vi "PC_Shot_PowerOG.vi"(5 "Bounce T/F?":bool, 7 "Puck Selection":enum32{"PTFE", "Nylon"}(radio), 8 "Error In":errorcluster, 11 "PC Data":T1) -> (0 "Error Out":errorcluster, 3 "Power %":dbl)   [LabVIEW 2017]
uses:
  pc_data.ctl
  <vilib>/vision/Image Controls.llb/IMAQ Image.ctl
  <vilib>/Utility/file.llb/Read Delimited Spreadsheet (DBL).vi
panel:
  out "Goal Y Straight":dbl
  in  "Friction PTFE":dbl=0.4
  in  "Puck Mass PTFE":dbl=0.0069
  in  "Friction Nylon":dbl=0.31
  in  "Puck Mass Nylon":dbl=0.0037
  out "mm/pixels":dbl
  out "Goal Y Bounce":dbl
  out "Wall X Bounce":dbl
  out "Pot Position":dbl
  out "Kicker angle":dbl
  in  "Pendulum length":dbl=0.069
  in  "Pendulum mass":dbl=0.096
  out "Required E":dbl
  in  "Kicker Res":dbl=0.5
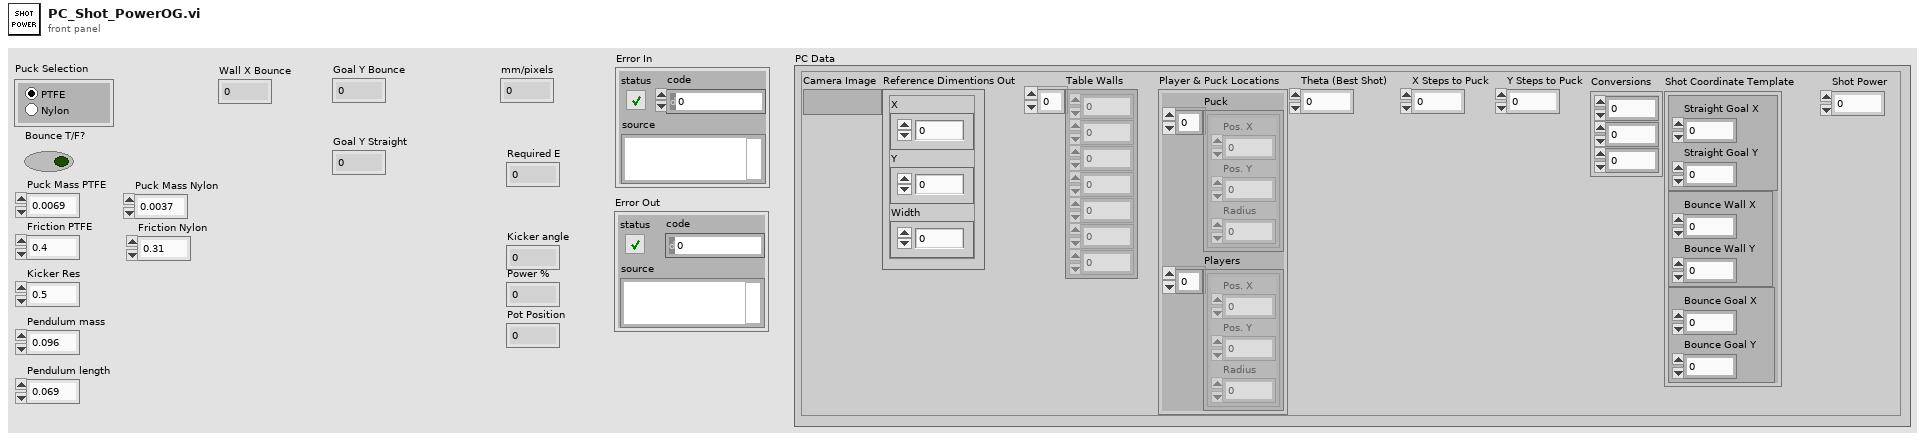
[diagram p1: front panel]
types:
  T1 = typedef "pc_data.ctl" = cluster{"Camera Image":T2, "Reference Dimentions Out":cluster{"X":dbl, "Y":dbl, "Width":dbl}, "Table Walls":sgl[], "Player & Puck Locations":cluster{"Puck":cluster{"Pos. X":i32, "Pos. Y":i32, "Radius":i32}[], "Players":cluster{"Pos. X":i32, "Pos. Y":i32, "Radius":i32}[]}, "Theta (Best Shot)":dbl, "X Steps to Puck":dbl, "Y Steps to Puck":dbl, "Conversions":cluster{dbl, dbl, dbl}, "Shot Coordinate Template":cluster{cluster{"Straight Goal X":sgl, "Straight Goal Y":dbl}, cluster{"Bounce Wall X":dbl, "Bounce Wall Y":sgl}, cluster{"Bounce Goal X":sgl, "Bounce Goal Y":dbl}}, "Shot Power":dbl}
  T2 = typedef "IMAQ Image.ctl" = refnum<image>
  T3 = cluster{"Pos. X":i32, "Pos. Y":i32, "Radius":i32}[]
  T4 = cluster{cluster{"Straight Goal X":sgl, "Straight Goal Y":dbl}, cluster{"Bounce Wall X":dbl, "Bounce Wall Y":sgl}, cluster{"Bounce Goal X":sgl, "Bounce Goal Y":dbl}}
  T5 = cluster{"Straight Goal X":sgl, "Straight Goal Y":dbl}
  T6 = cluster{"Bounce Wall X":dbl, "Bounce Wall Y":sgl}
  T7 = cluster{"Bounce Goal X":sgl, "Bounce Goal Y":dbl}
  T8 = cluster{"Pos. X":i32, "Pos. Y":i32, "Radius":i32}
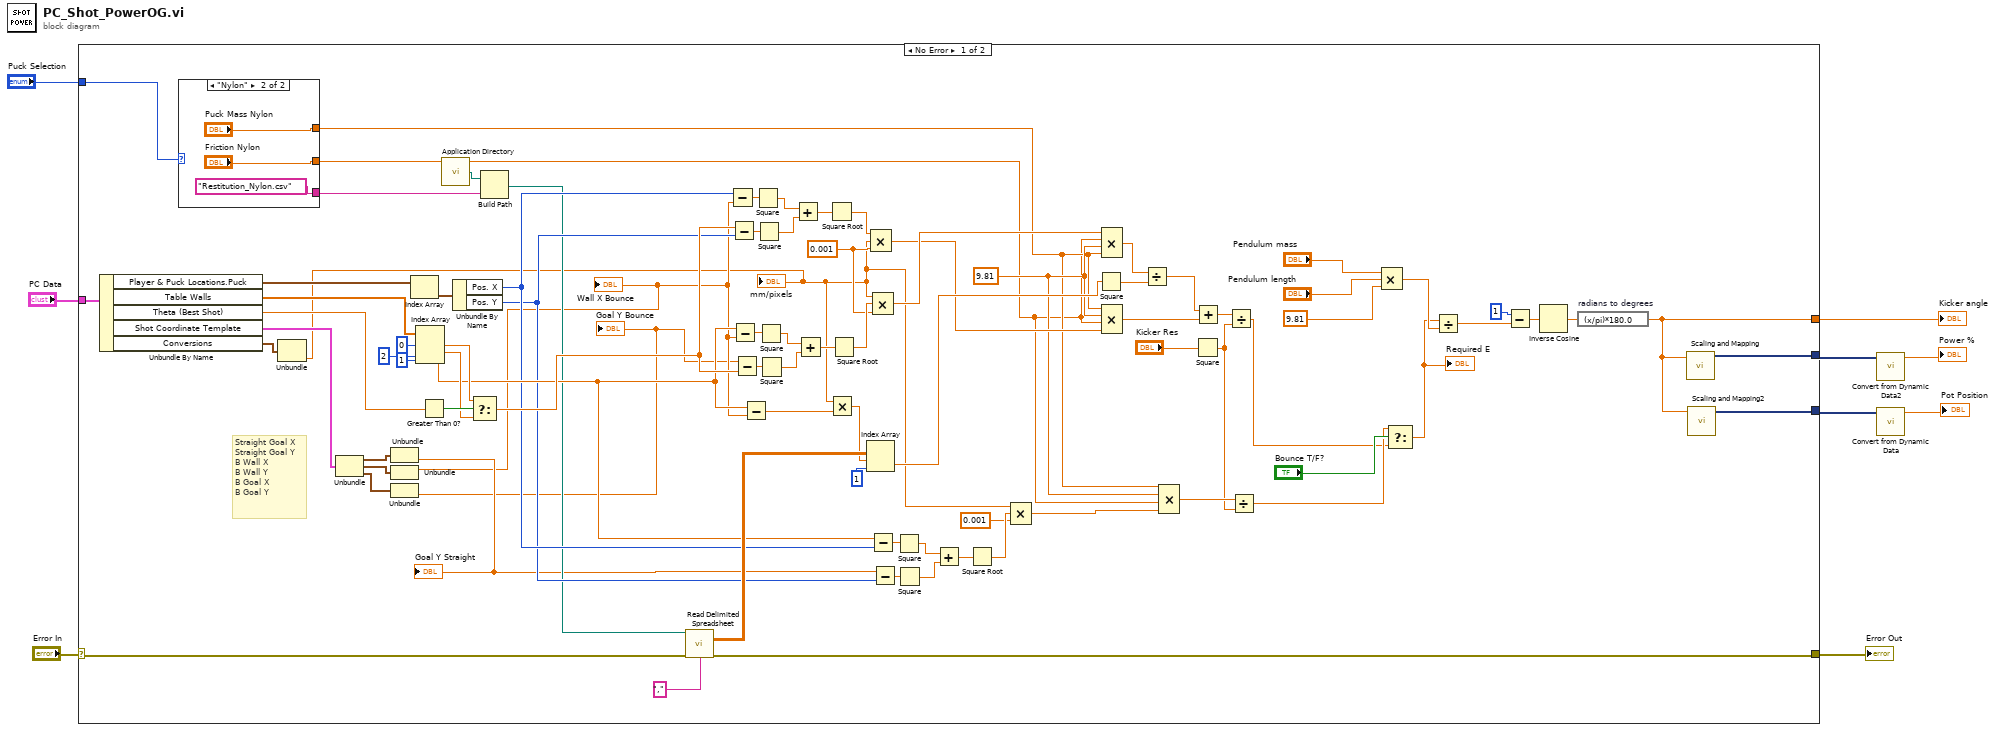
[diagram p0: block diagram]
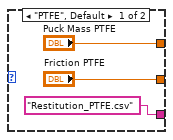
[diagram p2: hidden frame]
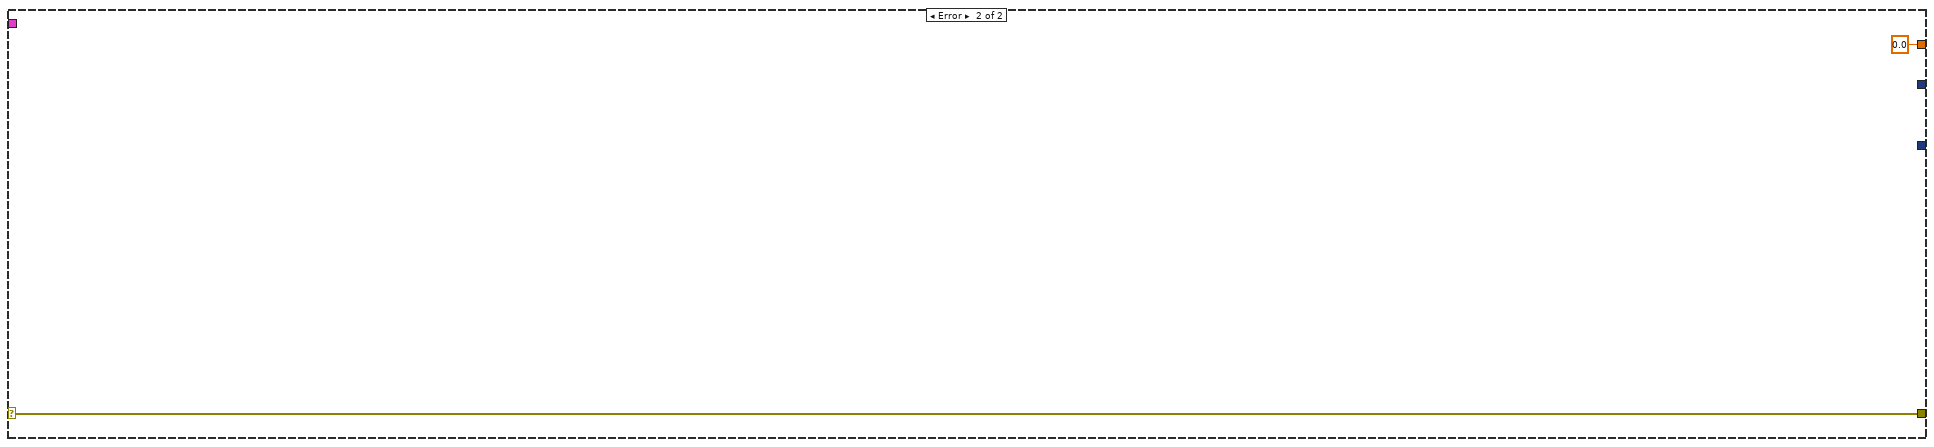
[diagram p3: hidden frame]
diagram:
  n1 = case shown="No Error" "Error In" {
    selector: "Error In" -> [w77 w102]
    tunnel: [w76 w102] -> w8
    tunnel: "Puck Selection" -> [w44 _]
    tunnel: "PC Data" -> [w28 _]
    tunnel: [w27 _] -> w1
    tunnel: [w26 _] -> w3
    tunnel: [w25 0.0] -> w5
    frame No Error {
      w48 = 0.001
      w58 = 9.81
      # "Straight Goal X\nStraight Goal Y\nB Wall X\nB Wall Y\nB Goal X\nB Goal Y"
      n2 = Unbundle By Name(w28) -> ("Player & Puck Locations.Puck"=w41:T3, "Table Walls"=w38:sgl[], "Theta (Best Shot)"=w21:dbl, "Shot Coordinate Template"=w20:T4, "Conversions"=w13:cluster{dbl, dbl, dbl})
      n3 = case shown="\"Nylon\"" w44 {
        tunnel: ["Puck Mass PTFE" "Puck Mass Nylon"] -> w43
        tunnel: ["Friction PTFE" "Friction Nylon"] -> w42
        tunnel: ["Restitution_PTFE.csv" "Restitution_Nylon.csv"] -> w22
        frame "PTFE", Default {
        }
        frame "Nylon" {
        }
      }
      n4 = Unbundle(w13) -> (w12:dbl)  [unwired: 2 out]
      "mm/pixels" <- w12
      n5 = Unbundle(w20) -> (w19:T5, w18:T6, w17:T7)
      n6 = Unbundle(w19) -> ("Straight Goal Y"=w16:dbl)  [unwired: 1 out]
      "Goal Y Straight" <- w16
      n7 = Unbundle(w18) -> ("Bounce Wall X"=w15:dbl)  [unwired: 1 out]
      "Wall X Bounce" <- w15
      n8 = Unbundle(w17) -> ("Bounce Goal Y"=w14:dbl)  [unwired: 1 out]
      "Goal Y Bounce" <- w14
      n9 = Index Array(array=w41) -> (element=w40:T8)  [unwired: 1 in]
      n10 = Index Array(array=w38, index #1=0 ("index"), index #2=2 ("index"), index #3=1 ("index")) -> (element #1=w35:sgl, element #2=w34:sgl, element #3=w31:sgl)
      n11 = Greater Than 0?(x=w21) -> (x > 0?=w39:bool)
      n12 = call <vilib>:"Application Directory.vi"() -> ("Application Directory"=w23:path)
      n13 = Unbundle By Name(w40) -> ("Pos. X"=w30:i32, "Pos. Y"=w29:i32)
      n14 = Select(t=w35, s=w39, f=w34) -> (s? t:f=w33:sgl)
      n15 = Build Path(base path=w23, name or relative path=w22) -> (appended path=w24:path)
      n16 = call-poly <vilib>:"Read Delimited Spreadsheet.vi"("file path (dialog if empty)"=w24, "error in (no error)"=w77, "delimiter (\\t)"="," ("delimiter (\\t)")) -> ("all rows"=w79:dbl[][], "error out"=w76:errorcluster)  [unwired: 7 in, 4 out]
      n17 = Subtract(x=w30, y=w15) -> (x-y=w74:dbl)
      n18 = Subtract(x=w33, y=w29) -> (x-y=w73:sgl)
      n19 = Subtract(x=w31, y=w15) -> (x-y=w69:dbl)
      n20 = Subtract(x=w14, y=w33) -> (x-y=w68:dbl)
      n21 = Subtract(x=w31, y=w15) -> (x-y=w46:dbl)
      n22 = Square(x=w74) -> (x^2=w71:dbl)
      n23 = Square(x=w73) -> (x^2=w72:sgl)
      n24 = Square(x=w69) -> (x^2=w66:dbl)
      n25 = Square(x=w68) -> (x^2=w67:dbl)
      n26 = Add(x=w71, y=w72) -> (x+y=w70:dbl)
      n27 = Add(x=w66, y=w67) -> (x+y=w65:dbl)
      n28 = Square Root(x=w70) -> (sqrt(x)=w64:dbl)
      n29 = Multiply(x=w12, y=w46) -> (x*y=w45:dbl)
      n30 = Square Root(x=w65) -> (sqrt(x)=w63:dbl)
      n31 = Index Array(array=w79, index (row)=w45, index (col)=1 ("disabled index (col)")) -> (element=w75:dbl)
      n32 = Subtract(x=w31, y=w30) -> (x-y=w52:sgl)
      n33 = Compound Arithmetic op=MULTIPLY(w64, w12, w48) -> (w61:dbl)
      n34 = Subtract(x=w16, y=w29) -> (x-y=w53:dbl)
      n35 = Compound Arithmetic op=MULTIPLY(w12, w63, w48) -> (w62:dbl)
      n36 = Square(x=w52) -> (x^2=w55:sgl)
      n37 = Square(x=w53) -> (x^2=w54:dbl)
      n38 = Add(x=w55, y=w54) -> (x+y=w56:dbl)
      n39 = Square Root(x=w56) -> (sqrt(x)=w57:dbl)
      n40 = Compound Arithmetic op=MULTIPLY(w12, w57, 0.001 ("value")) -> (w51:dbl)
      n41 = Square(x=w75) -> (x^2=w93:dbl)
      n42 = Compound Arithmetic op=MULTIPLY(w62, w42, w58, w43) -> (w94:dbl)
      n43 = Compound Arithmetic op=MULTIPLY(w43, w58, w42, w61) -> (w91:dbl)
      n44 = Divide(x=w94, y=w93) -> (x/y=w92:dbl)
      n45 = Compound Arithmetic op=MULTIPLY(w43, w58, w42, w51) -> (w50:dbl)
      n46 = Square(x="Kicker Res") -> (x^2=w49:dbl)
      n47 = Add(x=w92, y=w91) -> (x+y=w89:dbl)
      n48 = Divide(x=w89, y=w49) -> (x/y=w10:dbl)
      n49 = Divide(x=w50, y=w49) -> (x/y=w11:dbl)
      n50 = Compound Arithmetic op=MULTIPLY("Pendulum mass", "Pendulum length", 9.81) -> (w85:dbl)
      n51 = Select(t=w11, s="Bounce T/F?", f=w10) -> (s? t:f=w60:dbl)
      "Required E" <- w60
      n52 = Divide(x=w60, y=w85) -> (x/y=w84:dbl)
      n53 = Subtract(x=1, y=w84) -> (x-y=w82:dbl)
      n54 = Inverse Cosine(1:w82) -> (0:w81:dbl)
      n55 = expression code="(x/pi)*180.0" "radians to degrees"(w81) -> (w25:dbl)
      n56 = call "Scaling and Mapping"("Signals"=w25) -> ("Scaled Signals"=w26:dynamicdata)  [unwired: 9 in, 1 out]
      n57 = call "Scaling and Mapping2"("Signals"=w25) -> ("Scaled Signals"=w27:dynamicdata)  [unwired: 9 in, 1 out]
    }
    frame Error {
    }
  }
  "Error Out" <- w8
  "Kicker angle" <- w5
  n58 = call "Convert from Dynamic Data2"("Dynamic Data Type"=w3) -> ("Scalar"=→"Power %":dbl)  [unwired: 3 in]
  n59 = call "Convert from Dynamic Data"("Dynamic Data Type"=w1) -> ("Scalar"=→"Pot Position":dbl)  [unwired: 3 in]
